vi "Lux Calculator.vi"(6 "B_coef":dbl=-0.444 format="%#_13g", 7 "R_coef":dbl=0.136 format="%#_13g", 8 "CPL":dbl, 9 "B'":dbl, 10 "G'":dbl, 11 "R'":dbl) -> (2 "LUX":dbl)   [LabVIEW 2014, in "AMS TS3472 Light Sensor.lvlib" / "AMS TCS3472.lvclass"]
uses:
  AMS TCS3472.lvclass
panel:
  out "x*y 2":dbl
  out "G\"":dbl
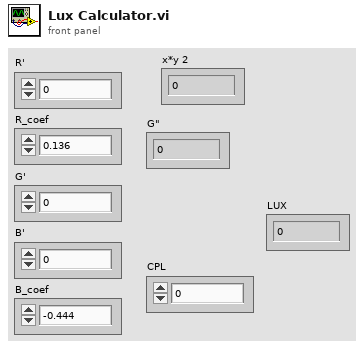
[diagram p1: front panel]
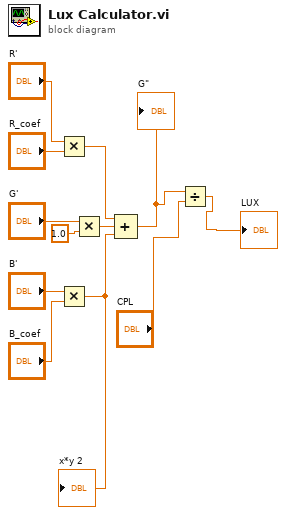
[diagram p0: block diagram]
diagram:
  n1 = Multiply(x="R'", y="R_coef") -> (x*y=w6:dbl)
  n2 = Multiply(x="B'", y="B_coef") -> (x*y=w4:dbl)
  "x*y 2" <- w4
  n3 = Multiply(x="G'", y=1.0) -> (x*y=w5:dbl)
  n4 = Compound Arithmetic op=ADD(w6, w5, w4) -> (w3:dbl)
  "G\"" <- w3
  n5 = Divide(x=w3, y="CPL") -> (x/y=→"LUX":dbl)
